vi "UI - All UI Objects Refs Memory - Get Reference - RadioButtonsControl.vi"(8 "error in (no error)":errorcluster, 10 "Variable In":string) -> (0 "error out":errorcluster, 2 "Found?":bool, 3 "Ref Out":refnum<vi>)   [LabVIEW 2012]
doc: "This VI will get the right reference (type) for UI objects that has already been initialized to the \"UI - All UI Objects Refs Memory.vi\" memory. So put that function to your MAIN VI and Use the INIT operation before you use this funtion.\n\n<B>Variable In:</B> This the UI object (control/indicator) label name that you want to control."
uses:
  Controls/UI - All UI Objects Refs Memory - Operation.ctl
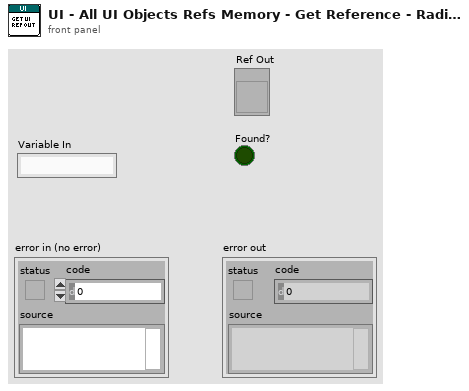
[diagram p1: front panel]
types:
  T1 = typedef "UI - All UI Objects Refs Memory - Operation.ctl" = enum16{"INIT", "GET", "ADD"}
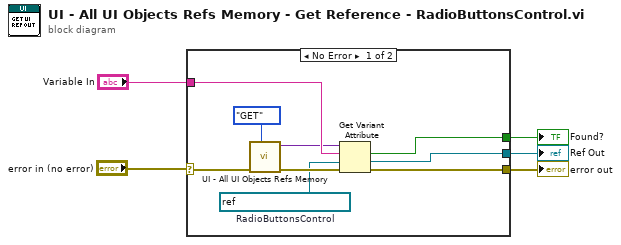
[diagram p0: block diagram]
diagram:
  n1 = case shown="No Error" "error in (no error)" {
    selector: "error in (no error)" -> [w10 w15]
    tunnel: [w13 w15] -> w5
    tunnel: "Variable In" -> [w14 _]
    tunnel: [w12 _] -> w2
    tunnel: [w11 _] -> w1
    frame No Error {
      w7 = refnum<vi> refnum  # RadioButtonsControl
      n2 = call "UI - All UI Objects Refs Memory.vi"("Operation"=UI_-_All_UI_Objects_Refs_Memory_-_Operation."GET", "error in"=w10) -> ("error out"=w9:errorcluster, "Variant Out"=w8:variant)  [unwired: 8 in]
      n3 = Get Variant Attribute(Variant=w8, name=w14, default value (empty Variant)=w7, error in=w9) -> (found=w12:bool, value=w11:refnum<vi>, error out=w13:errorcluster)  [unwired: 1 out]
    }
    frame Error {
    }
  }
  "error out" <- w5
  "Found?" <- w2
  "Ref Out" <- w1
